vi "Planing Set.vi"(8 "error in (no error)":errorcluster, 9 "Planing":bool=TRUE, 10 "Reset":bool) -> (0 "error out":errorcluster, 2 "Number of Clicks":i8)   [LabVIEW 2021, in "Haptic Prog Interface.lvlib"]
doc: "Returns the horizontal xy-position of the haptic pen in nm, and the vertical z-position in mm. The horizontal position depends on the frame origin and frame size.\n\n<b>Position:</b> Returns a cluster of the x (nm), y (nm), and z (mm) positions of the pen."
uses:
  Haptic Prog Interface.lvlib
  Haptic-Programming-Interface/src/x64/Debug/Haptic Programming Interface.dll
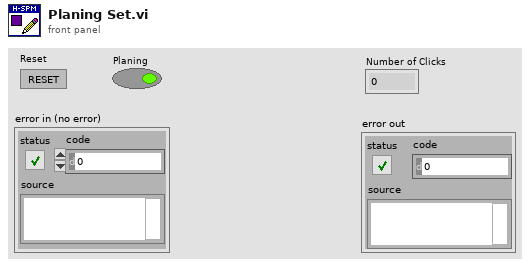
[diagram p1: front panel]
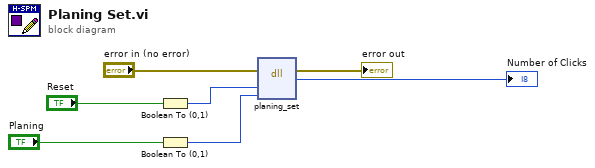
[diagram p0: block diagram]
diagram:
  n1 = Boolean To (0,1)(Boolean="Reset") -> (0, 1=w5:i16)
  n2 = Boolean To (0,1)(Boolean="Planing") -> (0, 1=w3:i16)
  n3 = dll-call lib="C:/Users/freem/Documents/GitHub/Haptic-Programming-Interface/src/x64/Debug/Haptic Programming Interface.dll" fn="planing_set"(error in="error in (no error)", "reset"=w5, "toggle"=w3) -> (error out=→"error out":errorcluster, "return type"=→"Number of Clicks":i8)  [unwired: 4 in, 1 out]
